vi "FindAddHandler.vi"(8 "ByNameOnly?":bool=TRUE, 9 "Extensions":string[](array[string]), 10 "Name":string, 11 "AddHandlers":T1[](array[typedef])) -> (2 "Found":bool, 3 "Index":i32)   [LabVIEW 2020]
uses:
  <vilib>/WebServerConfig/AddHandler.ctl
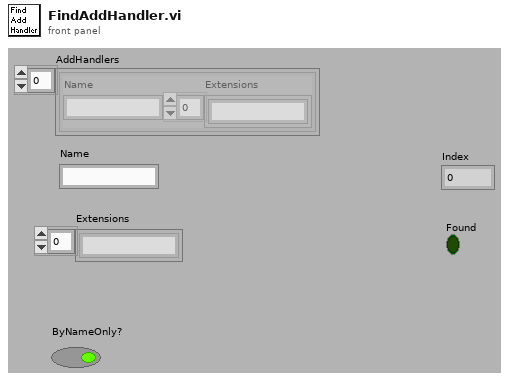
[diagram p1: front panel]
types:
  T1 = typedef "AddHandler.ctl" = cluster{"Name":string, "Extensions":string[]}
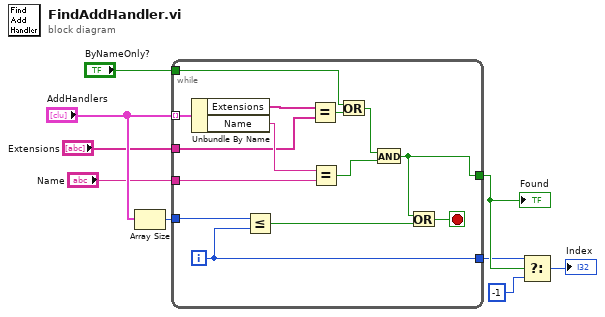
[diagram p0: block diagram]
diagram:
  n1 = Array Size(array="AddHandlers") -> (size(s)=w8:i32)
  n2 = while {
    tunnel: w8 -> [w23]
    tunnel: "AddHandlers" -> [w20] mode=indexing
    tunnel: [w14] -> w6
    tunnel: [w19] -> w5
    tunnel: "ByNameOnly?" -> [w18]
    tunnel: "Extensions" -> [w10]
    tunnel: "Name" -> [w11]
    i -> [w19]
    stop <- w21 stop-if-true
    n3 = Unbundle By Name(w20) -> ("Extensions"=w13:string[], "Name"=w12:string)
    n4 = Less Or Equal?(x=w23, y=w19) -> (x <= y?=w22:bool)
    n5 = Equal?(x=w13, y=w10) -> (x = y?=w17:bool)
    n6 = Equal?(x=w12, y=w11) -> (x = y?=w15:bool)
    n7 = Or(x=w18, y=w17) -> (x .or. y?=w16:bool)
    n8 = And(x=w16, y=w15) -> (x .and. y?=w14:bool)
    n9 = Or(x=w14, y=w22) -> (x .or. y?=w21:bool)
  }
  "Found" <- w6
  n10 = Select(t=w5, s=w6, f=-1) -> (s? t:f=→"Index":i32)
